vi "set design tool filepaths.vi"(2 "error in (no error)":errorcluster) -> (0 "error out":errorcluster, 1 "Success":bool)   [LabVIEW 2015]
uses:
  <vilib>/Utility/config.llb/NI_LVConfig.lvlib
  Instance           3 33Saved   set design tool filepaths .vi
  <vilib>/Utility/config.llb/Write Key (Path).vi
  <vilib>/Utility/config.llb/Read Key (Boolean).vi
  Folders.ctl
panel:
  out "application name":string
  out "Prompt":string[](array[string])
  out "Key":string[](array[string])
  in  "Folders":T1
  # "3 folders\nFInal Designs\nFolder with incoming requests\nFolder with completed designs"
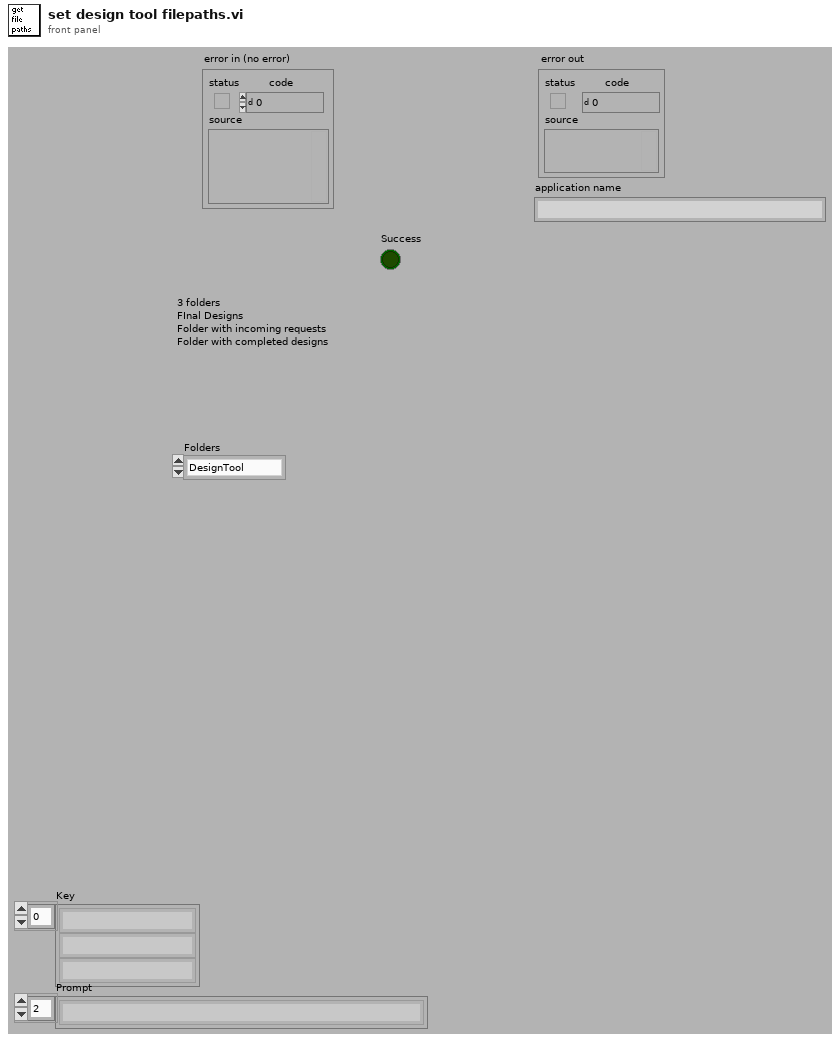
[diagram p1: front panel]
types:
  T1 = typedef "Folders.ctl" = enum16{"DesignTool", "RequestedDesigns", "CompletedDesigns"}
  T2 = typedef "NI_LVConfig.lvlib/Config Data RefNum.ctl" = refnum<k1>
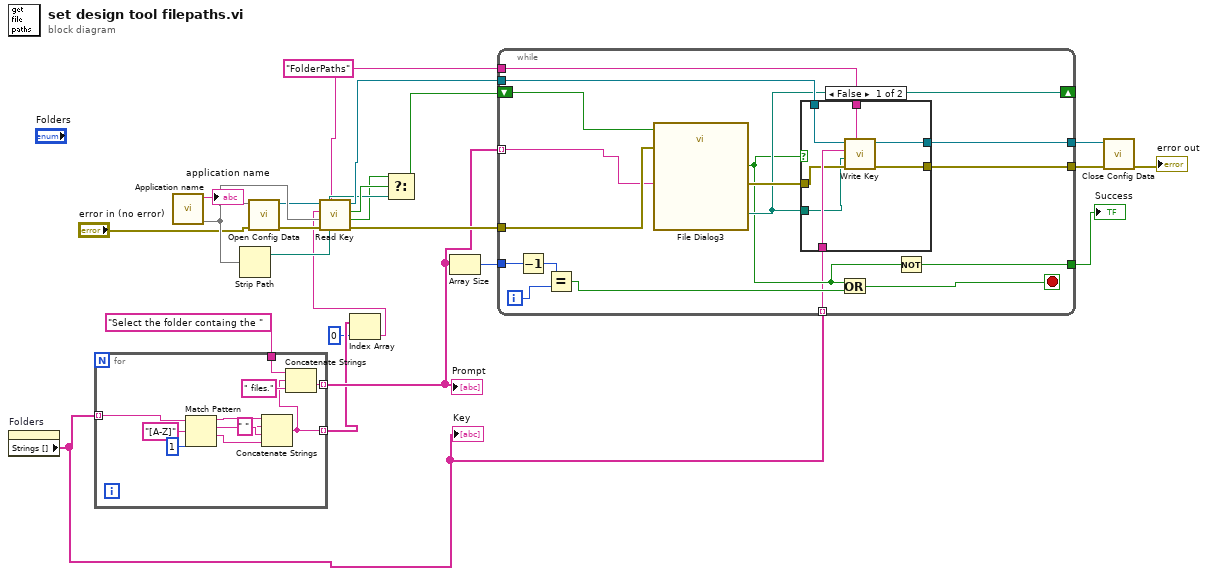
[diagram p0: block diagram]
diagram:
  w8 = "FolderPaths" ("section")
  n1 = property on="Folders" class="Enum (strict)"() -> ("Strings []"=w1:string[])  [unwired: 2 in, 2 out]
  "Key" <- w1
  n2 = for {
    tunnel: w1 -> [w34] mode=indexing
    tunnel: [w24] -> w5 mode=indexing
    tunnel: "Select the folder containg the " -> [w27]
    tunnel: [w25] -> w6 mode=indexing
    n3 = Match Pattern(string=w34, regular expression="[A-Z]", offset (0)=1) -> (before substring=w32:string, match substring=w31:string, after substring=w30:string)  [unwired: 1 out]
    n4 = Concatenate Strings(w32, " " ("string"), w31, w30) -> (w24:string)
    n5 = Concatenate Strings(w27, w24, " files." ("string")) -> (w25:string)
  }
  "Prompt" <- w6
  n6 = call "Application name.vi"() -> (0:w22, "application name"=→"application name":string)  [unwired: 4 in, 2 out]
  n7 = Strip Path(path=w22) -> (stripped path=w13:path)  [unwired: 1 out]
  n8 = call <vilib>:"Open Config Data.vi"("error in (no error)"="error in (no error)", "configuration file path"=w22) -> ("error out"=w20:errorcluster, "refnum"=w21:T2)  [unwired: 7 in, 1 out]
  n9 = Index Array(array=w5, index=0) -> (element=w3:string)
  n10 = call-poly <vilib>:"Read Key.vi"("section"=w8, "error in (no error)"=w20, "default value"=w22, "key"=w3, "refnum"=w21) -> ("error out"=w17:errorcluster, "value"=w12:bool, "found?"=w23:bool, "refnum out"=w18:T2)  [unwired: 3 in]
  n11 = Select(t=w12, s=w23, f=w13) -> (s? t:f=w11:bool)
  n12 = Array Size(array=w6) -> (size(s)=w10:i32)
  n13 = while {
    tunnel: w6 -> [w36] mode=indexing
    shift-right: [w45] -> _
    shift-left: w11 -> [w44]
    tunnel: w18 -> [w51]
    tunnel: w8 -> [w50]
    tunnel: w17 -> [w48]
    tunnel: [w47] -> w15
    tunnel: [w46] -> w14
    tunnel: w10 -> [w42]
    tunnel: [w37] -> w9
    tunnel: w1 -> [w35] mode=indexing
    i -> [w40]
    stop <- w43 stop-if-true
    n14 = Decrement(x=w42) -> (x-1=w41:i32)
    n15 = Equal?(x=w41, y=w40) -> (x = y?=w39:bool)
    n16 = call "File Dialog3"("start path"=w44, "prompt"=w36, "error in"=w48) -> ("selected path"=w45:path, "cancelled"=w38:bool, "error out"=w49:errorcluster)  [unwired: 9 in, 1 out]
    n17 = case shown="False" w38 {
      tunnel: w51 -> [w58 w59]
      tunnel: w35 -> [w57 _]
      tunnel: w50 -> [w56 _]
      tunnel: w49 -> [w55 w60]
      tunnel: [w54 w59] -> w47
      tunnel: [w53 w60] -> w46
      tunnel: w45 -> [w52 _]
      frame False {
        n18 = call-poly <vilib>:"Write Key.vi"("section"=w56, "error in (no error)"=w55, "value"=w52, "key"=w57, "refnum"=w58) -> ("error out"=w53:errorcluster, "refnum out"=w54:T2)  [unwired: 4 in, 1 out]
      }
      frame True {
      }
    }
    n19 = Or(x=w38, y=w39) -> (x .or. y?=w43:bool)
    n20 = Not(x=w38) -> (.not. x?=w37:bool)
  }
  "Success" <- w9
  n21 = call <vilib>:"Close Config Data.vi"("error in (no error)"=w14, "refnum"=w15) -> ("error out"=→"error out":errorcluster)  [unwired: 8 in, 1 out]
